vi "Tarea de Control Avanzado correcto.vi"() -> ()   [LabVIEW 2020]
uses:
  <vilib>/addons/Control Design/_Model Construction/Data Typedefs.llb/CD Time Info.ctl
  <vilib>/imath/engines/lvmath2/RunTimeSupport/NIMS_Get Any Vector_w Error - Matrix.vi
  <instcachedir>/0/NIMS_Get Any Vector_w Error - Matrix_03E716A238FA4CA1B10D931DADE97109.lvgen/NIMS_Get Any Vector_w Error - Matrix_03E716A238FA4CA1B10D931DADE97109_001.vi
  <vilib>/imath/engines/lvmath2/RunTimeSupport/NIMS_Get Scalar_w Error.vi
  <instcachedir>/0/NIMS_Get Scalar_w Error_5A0E401CB6154DCF81784DB8E431B6E1.lvgen/NIMS_Get Scalar_w Error_5A0E401CB6154DCF81784DB8E431B6E1_010.vi
  <vilib>/imath/engines/lvmath2/RunTimeEngine/BuiltInFunctions/ss_to_tf/NIMS_ss_to_tf(4i).vi
  <vilib>/imath/engines/lvmath2/RunTimeEngine/ErrorHandling/NIMS_Create Error From Enums.vi
  <vilib>/imath/engines/lvmath/Plug In/Control Design/BuiltInFunctions/tf/NIMS_CD_tf(num,den,Ts).vi
  <vilib>/imath/engines/lvmath/Plug In/Control Design/BuiltInFunctions/ackermann/NIMS_CD_ackermann(A,B,poles,STR).vi
  <vilib>/imath/engines/lvmath2/RunTimeEngine/ArithmeticOperatorToken/NIMS_ArithmeticOperator_power(S).vi
  <instcachedir>/0/NIMS_ArithmeticOperator_power(S)_0FB4C2FA3CD746849DC4699515FAC284.lvgen/NIMS_ArithmeticOperator_power(S)_0FB4C2FA3CD746849DC4699515FAC284_010.vi
  <vilib>/imath/engines/lvmath2/RunTimeEngine/BuiltInFunctions/abs/NIMS_abs(signed).vi
  <instcachedir>/0/NIMS_abs(signed)_C4FCB8E6058B49B797C7C8D53CA5F6EC.lvgen/NIMS_abs(signed)_C4FCB8E6058B49B797C7C8D53CA5F6EC_002.vi
  <vilib>/imathl/engines/lvmath/Functions/Error Handling/Create Error.vi
  <vilib>/imath/engines/lvmath2/RunTimeEngine/BuiltInFunctions/roots/NIMS_roots.vi
  <instcachedir>/0/NIMS_roots_5371068BAABD481CB00E0B78F1D2DC4F.lvgen/NIMS_roots_5371068BAABD481CB00E0B78F1D2DC4F_001.vi
  <vilib>/imath/engines/lvmath2/RunTimeEngine/ArithmeticOperatorToken/NIMS_ArithmeticOperator_multmx.vi
  <instcachedir>/0/NIMS_ArithmeticOperator_multmx_177F0753FB7A49B190E35F5DD0E80316.lvgen/NIMS_ArithmeticOperator_multmx_177F0753FB7A49B190E35F5DD0E80316_004.vi
  <vilib>/imath/engines/lvmath2/RunTimeEngine/ArithmeticOperatorToken/NIMS_ArithmeticOperator_minus.vi
  <instcachedir>/0/NIMS_ArithmeticOperator_minus_822089A08BE049DB927E6BEA78E100F1.lvgen/NIMS_ArithmeticOperator_minus_822089A08BE049DB927E6BEA78E100F1_002.vi
  <vilib>/imath/engines/lvmath2/RunTimeEngine/NodeEndStatement/NIMS_NodeEndStatement_Output.vi
  <instcachedir>/0/NIMS_NodeEndStatement_Output_53EC0D466D134D7ABD903AC30B43404B.lvgen/NIMS_NodeEndStatement_Output_53EC0D466D134D7ABD903AC30B43404B_000.vi
  <instcachedir>/0/NIMS_NodeEndStatement_Output_53EC0D466D134D7ABD903AC30B43404B.lvgen/NIMS_NodeEndStatement_Output_53EC0D466D134D7ABD903AC30B43404B_010.vi
  <instcachedir>/0/NIMS_NodeEndStatement_Output_53EC0D466D134D7ABD903AC30B43404B.lvgen/NIMS_NodeEndStatement_Output_53EC0D466D134D7ABD903AC30B43404B_005.vi
  <vilib>/imath/engines/lvmath2/RunTimeEngine/ErrorHandling/NIMS_Finalize Error.vi
  <vilib>/addons/Control Design/_Time Response Analysis/Time Response.llb/Time Response subVI/cd_Step Response (Transfer Function).vi
  <vilib>/addons/Control Design/_Dynamic Analysis/Dynamic Analysis.llb/Dynamic Analysis subVI/cd_Poles (Transfer Function).vi
  <vilib>/addons/Control Design/_Utility/Model Viewer.llb/Model Viewer SubVI/cd_Draw Transfer Function Equation (TF).vi
  <vilib>/addons/Control Design/_Dynamic Analysis/Dynamic Analysis.llb/Dynamic Analysis subVI/cd_Root Locus (Transfer Function).vi
  <vilib>/addons/Control Design/_Model Conversions/Model Type.llb/Model Conversion SubVI/cd_Convert Transfer Function to State-Space Model.vi
  <vilib>/addons/Control Design/_Utility/Model Viewer.llb/Model Viewer SubVI/cd_Draw Zero-Pole-Gain Equation (TF).vi
  <vilib>/addons/Control Design/_Utility/NI_CD_Model Viewer.lvlib
  <vilib>/addons/Control Design/_Model Construction/NI_LinSys_Data Typedefs.lvlib
  <vilib>/addons/Control Design/_Dynamic Analysis/NI_CD_Dynamic Analysis.lvlib
  <vilib>/addons/Control Design/_State-Space Analysis/NI_CD_State-Space Analysis.lvlib
  <vilib>/addons/Control Design/_Model Conversions/NI_CD_Model Type.lvlib
  <vilib>/addons/Control Design/_Time Response Analysis/NI_CD_Time Response.lvlib
panel:
  in  "D":dbl[](array[numeric])
  in  "B":dbl[][](array[numeric])
  out "Root Locus Data":cluster{"K":dbl[], "Roots":cdb[][]} {"Roots" format="%.4f"; "K" format="%.4g"}
  out "Root Locus Graph":cluster{dbl[], dbl[]}[](graph)
  out "Is Observable?":bool
  out "Observability  Matrix":dbl[][](array[numeric]) format="%#.2g"
  out "Is Stabilizable?":bool
  out "Is Controllable?":bool
  out "Controllability Matrix":dbl[][](array[numeric])=[[1.0, 0.0, 6.0], [0.0, 1.0, -1.0], [0.0, 0.0, 0.0]] format="%.2f"
  out "Poles":cdb[](array[numeric]) format="%.2f"
  out "Equation 2":picture
  out "K1":dbl[](array[numeric])
  out "Pd":cdb[](array[numeric])
  out "Equation 3":picture
  out "Equation":picture
  in  "Polos Propuestos":cdb[](array[numeric])=[0.0+0.0i, 1.0+0.0i, 0.0+0.0i]
  in  "C":dbl[](array[numeric])=[0.0, 1.0, 0.0]
  in  "A":dbl[][](array[numeric])=[[0.0, 1.0, 0.0], [0.0, 0.0, 1.0], [0.0, -2.0, -3.0]]
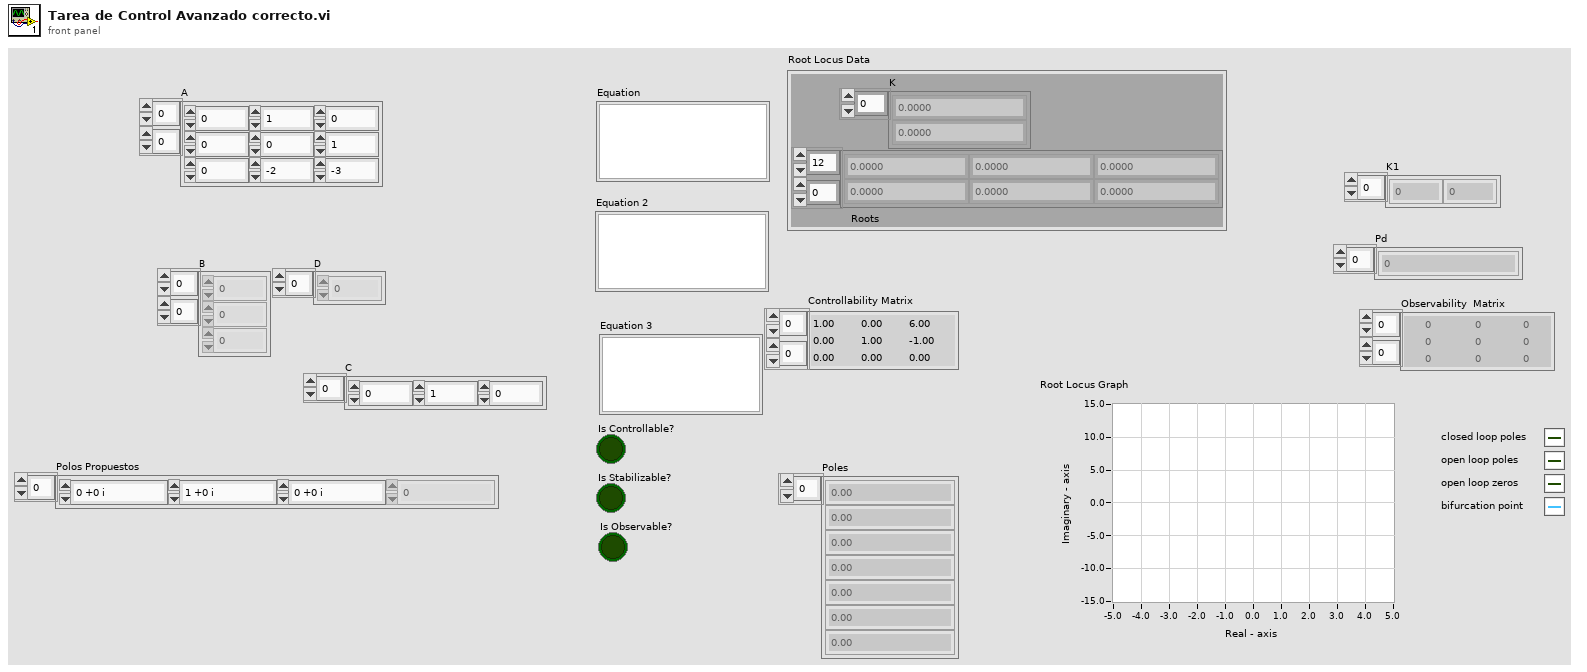
[diagram p1: front panel]
types:
  T1 = typedef "NI_LinSys_Data Typedefs.lvlib/CD Time Info.ctl" = cluster{"t0":dbl, "dt":dbl, "tf":dbl}
  T2 = typedef "NI_LinSys_Model Typedefs.lvlib/CD Transfer Function Model (MIMO).ctl" = cluster{"properties":T3, "transfer function(s)":T4[][]}
  T3 = typedef "NI_LinSys_Model Typedefs.lvlib/CD General Elements.ctl" = cluster{"Model name":string, "Input names":string[], "Output names":string[], "Input Delays":dbl[], "Output Delays":dbl[], "Sampling Time":dbl, "Notes":string}
  T4 = typedef "NI_LinSys_Model Typedefs.lvlib/CD Transfer Function Model (SISO).ctl" = cluster{"Numerator":dbl[], "Denominator":dbl[], "delay":dbl}
  T5 = typedef "NI_LinSys_Model Typedefs.lvlib/CD State Space Model (MIMO).ctl" = cluster{"properties":T3, "A":dbl[][], "B":dbl[][], "C":dbl[][], "D":dbl[][], "StateNames":string[], "Transport Delay":dbl[][]}
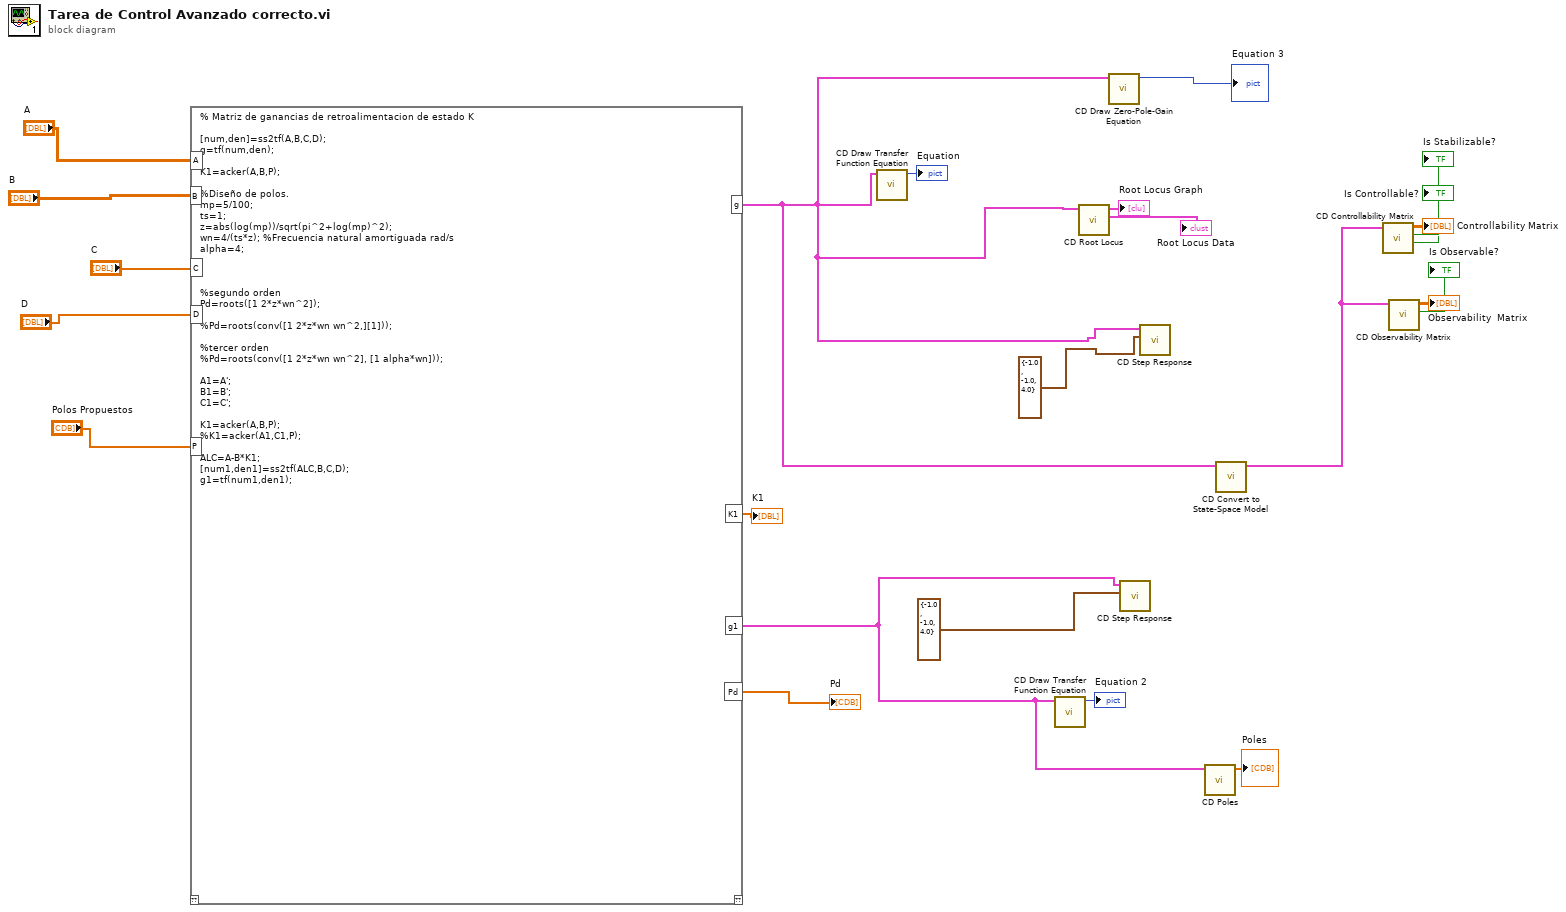
[diagram p0: block diagram]
diagram:
  n1 = mathscript code="% Matriz de ganancias de retroalimentacion de estado K\n\n[num,den]=ss2tf(A,B,C,D);\ng=tf(num,den);\n\nK1=acker(A,B,P);\n\n%Diseño de polos.\nmp=5/100;\nts=1;\nz=abs(log(mp))/sqrt(pi^2+log(mp)^2);\nwn=4/(ts*z); %Frecuencia natural amortiguada rad/s\nalpha=4;\n\n\n\n%segundo orden\nPd=roots([1 2*z*wn^2]);\n\n%Pd=roots(conv([1 2*z*wn wn^2,][1]));\n\n%tercer orden\n%Pd=roots(conv([1 2*z*wn wn^2], [1 alpha*wn]));\n\nA1=A';\nB1=B';\nC1=C';\n\nK1=acker(A,B,P);\n%K1=acker(A1,C1,P);\n\nALC=A-B*K1;\n[num1,den1]=ss2tf(ALC,B,C,D);\ng1=tf(num1,den1);"("B"="B", "C"="C", "D"="D", "P"="Polos Propuestos", "A"="A") -> ("g"=w4:T2, "K1"=→"K1":dbl[], "g1"=w7:T2, "Pd"=→"Pd":cdb[])  [unwired: 1 in, 1 out]
  n2 = call-poly <vilib>:"CD Draw Transfer Function Equation.vi"("Transfer Function Model"=w4) -> ("Equation"=→"Equation":picture)  [unwired: 8 in, 2 out]
  n3 = call-poly <vilib>:"CD Draw Transfer Function Equation.vi"("Transfer Function Model"=w7) -> ("Equation"=→"Equation 2":picture)  [unwired: 8 in, 2 out]
  n4 = call-poly <vilib>:"CD Root Locus.vi"("Transfer Function Model"=w4) -> ("Root Locus Data"=→"Root Locus Data":cluster{"K":dbl[], "Roots":cdb[][]}, "Root Locus Graph"=→"Root Locus Graph":cluster{dbl[], dbl[]}[])  [unwired: 7 in, 2 out]
  n5 = call-poly <vilib>:"CD Draw Zero-Pole-Gain Equation.vi"("Transfer Function Model"=w4) -> ("Equation"=→"Equation 3":picture)  [unwired: 8 in, 2 out]
  n6 = call-poly <vilib>:"CD Step Response.vi"("Time Range"=T1 {"t0"=-1.0, "dt"=-1.0, "tf"=4.0}, "Transfer Function Model"=w7) -> ()  [unwired: 7 in, 3 out]
  n7 = call-poly <vilib>:"CD Step Response.vi"("Time Range"=T1 {"t0"=-1.0, "dt"=-1.0, "tf"=4.0}, "Transfer Function Model"=w4) -> ()  [unwired: 7 in, 3 out]
  n8 = call-poly <vilib>:"CD Poles.vi"("Transfer Function Model"=w7) -> ("Poles"=→"Poles":cdb[])  [unwired: 9 in, 1 out]
  n9 = call-poly <vilib>:"CD Convert to State-Space Model.vi"("Transfer Function Model"=w4) -> ("State-Space Model"=w15:T5)  [unwired: 9 in, 1 out]
  n10 = call <vilib>:"CD Controllability Matrix.vi"("State-Space Model"=w15) -> ("Is Stabilizable?"=→"Is Stabilizable?":bool, "Is Controllable?"=→"Is Controllable?":bool, "Controllability Matrix"=→"Controllability Matrix":dbl[][])  [unwired: 7 in, 1 out]
  n11 = call <vilib>:"CD Observability Matrix.vi"("State-Space Model"=w15) -> ("Is Observable?"=→"Is Observable?":bool, "Observability  Matrix"=→"Observability  Matrix":dbl[][])  [unwired: 7 in, 2 out]
